vi "MLP simple.vi"() -> ()   [LabVIEW 2015]
uses:
  <vilib>/Analysis/baseanly.llb/Real A x B.vi
  <vilib>/Analysis/NI_AALBase.lvlib
panel:
  out "Image Classes":i32[](array[numeric])
  out "Character Images":picture[](array[picture])
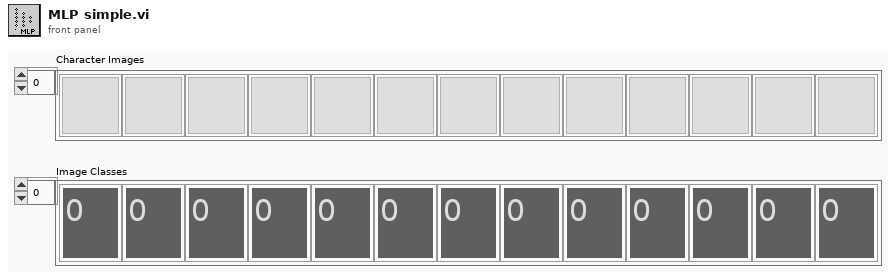
[diagram p1: front panel]
types:
  T1 = typedef "NI_Matrix.lvlib/RealMatrix.ctl" = dbl[][]
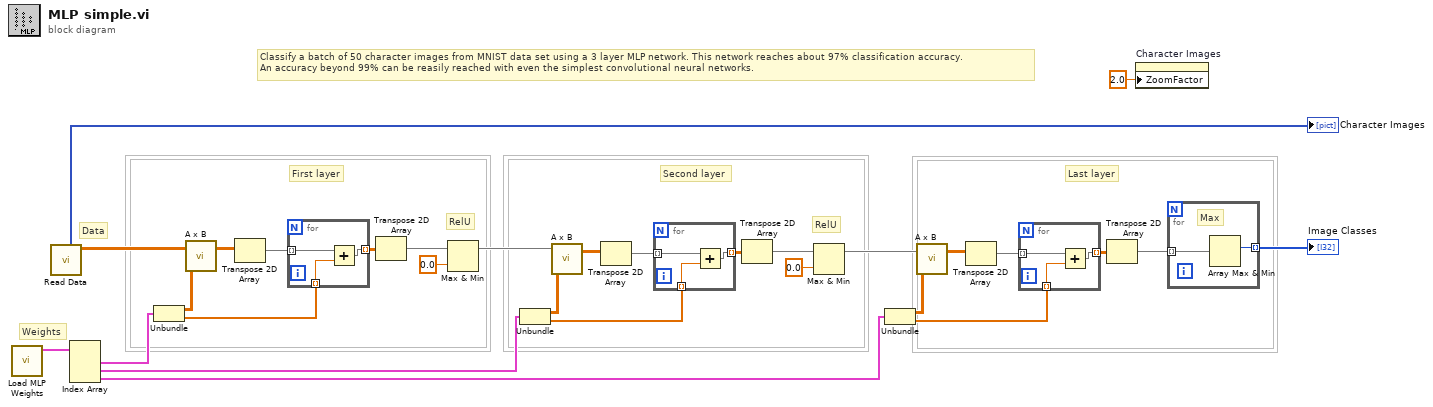
[diagram p0: block diagram]
diagram:
  # "Second layer"
  # "RelU"
  # "RelU"
  # "Last layer"
  # "Data"
  # "Weights"
  # "Classify a batch of 50 character images from MNIST data set using a 3 layer MLP network. This network reaches about 97% classification accuracy.\nAn accuracy beyond 99% can be reasily reached with even the simplest convolutional neural networks."
  # "First layer"
  n1 = call "Load MLP Weights.vi"() -> ("Weights"=w14:cluster{"Weights":dbl[][], "Biases":dbl[]}[])  [unwired: 10 in, 1 out]
  n2 = call "Read Data.vi"() -> ("Normalized Data"=w29:dbl[][], "Character Images"=→"Character Images":picture[])  [unwired: 9 in, 1 out]
  n3 = Index Array(array=w14) -> (element #1=w13:cluster{"Weights":dbl[][], "Biases":dbl[]}, element #2=w11:cluster{"Weights":dbl[][], "Biases":dbl[]}, element #3=w5:cluster{"Weights":dbl[][], "Biases":dbl[]})  [unwired: 3 in]
  n4 = Unbundle(w13) -> ("Weights"=w28:dbl[][], "Biases"=w23:dbl[])
  n5 = call-poly <vilib>:"A x B.vi"("B"=w28, "A"=w29) -> ("A x B"=w26:T1)  [unwired: 1 out]
  n6 = Transpose 2D Array(2D array=w26) -> (transposed array=w27:T1)
  n7 = for {
    tunnel: [w33] -> w25 mode=indexing
    tunnel: w27 -> [w32] mode=indexing
    tunnel: w23 -> [w31] mode=indexing
    n8 = Add ("Add.vi")(x=w32, y=w31) -> (x+y=w33:dbl[])
  }
  n9 = Transpose 2D Array(2D array=w25) -> (transposed array=w24:dbl[][])
  n10 = Max & Min(x=w24, y=0.0 ("f")) -> (max(x,y)=w12:dbl[][])  [unwired: 1 out]
  n11 = Unbundle(w11) -> ("Weights"=w15:dbl[][], "Biases"=w20:dbl[])
  n12 = call-poly <vilib>:"A x B.vi"("B"=w15, "A"=w12) -> ("A x B"=w17:T1)  [unwired: 1 out]
  n13 = Transpose 2D Array(2D array=w17) -> (transposed array=w16:T1)
  n14 = for {
    tunnel: [w36] -> w18 mode=indexing
    tunnel: w16 -> [w35] mode=indexing
    tunnel: w20 -> [w34] mode=indexing
    n15 = Add ("Add.vi")(x=w35, y=w34) -> (x+y=w36:dbl[])
  }
  n16 = Transpose 2D Array(2D array=w18) -> (transposed array=w19:dbl[][])
  n17 = Max & Min(x=w19, y=0.0 ("f")) -> (max(x,y)=w4:dbl[][])  [unwired: 1 out]
  n18 = Unbundle(w5) -> ("Weights"=w6:dbl[][], "Biases"=w10:dbl[])
  n19 = call-poly <vilib>:"A x B.vi"("B"=w6, "A"=w4) -> ("A x B"=w8:T1)  [unwired: 1 out]
  n20 = Transpose 2D Array(2D array=w8) -> (transposed array=w7:T1)
  n21 = for {
    tunnel: [w39] -> w9 mode=indexing
    tunnel: w7 -> [w38] mode=indexing
    tunnel: w10 -> [w37] mode=indexing
    n22 = Add ("Add.vi")(x=w38, y=w37) -> (x+y=w39:dbl[])
  }
  n23 = Transpose 2D Array(2D array=w9) -> (transposed array=w3:dbl[][])
  n24 = property on="Character Images" class="Pict"("ZoomFactor"=sgl 2.0 ("Zoom Factor")) -> ()  [unwired: 2 in, 2 out]
  n25 = for {
    tunnel: w3 -> [w40] mode=indexing
    tunnel: [w41] -> w2 mode=indexing
    # "Max"
    n26 = Array Max & Min(array=w40) -> (max index (indices)=w41:i32)  [unwired: 3 out]
  }
  "Image Classes" <- w2
